vi "DTFDcontroller.vi"() -> ()   [LabVIEW 2020]
uses:
  <vilib>/rvi/Analysis/control/linear/templates/niFPGA FXP Transfer Function Model.ctl
  <vilib>/Platform/TimedLoop/XDataNode/timing_clust.ctl
  <vilib>/Platform/TimedLoop/XDataNode/nitl_modes.ctl
  <vilib>/Platform/TimedLoop/XDataNode/wakeup.ctl
  <vilib>/rvi/Emulation/niFpgaSctlEmulationGetInTimedLoop.vi
  <vilib>/rvi/Emulation/niFpgaEmulationReportErrorSimple.vi
  <vilib>/rvi/Emulation/niFpgaGetClockAttributes.vi
  <vilib>/rvi/Emulation/niFpgaCriticalErrorInLSC.vi
  <vilib>/Platform/TimedLoop/XDataNode/XDataNode.xnode
  <vilib>/Platform/TimedLoop/XDataNode/XDNodeRunTimeDep.lvlib
panel:
  in  "H2 coefficients":T1={"Numerator"=[0.0, 0.0, 0.0, 0.0, 0.0, 0.0, 0.0, 0.0, 0.0], "Denominator"=[0.0, 0.0, 0.0, 0.0, 0.0, 0.0, 0.0, 0.0, 0.0], "Order"=0}
  in  "H1 coefficients":T1={"Numerator"=[0.0, 0.0, 0.0, 0.0, 0.0, 0.0, 0.0, 0.0, 0.0], "Denominator"=[0.0, 0.0, 0.0, 0.0, 0.0, 0.0, 0.0, 0.0, 0.0], "Order"=0}
  in  "KiTs":fxp<+,11,-22>=1.25030055642128e-07 format="%#_61g"
  in  "Kp":fxp<+/-,32,-4>
  in  "min":fxp<+/-,15,-7>=-0.003301858901977539 format="%#_50g"
  in  "max":fxp<+,15,-8>=0.00330197811126709 format="%#_51g"
  in  "Kp_Spool_2":fxp<+,3,4>=10.0 format="%#_20g"
  out "I_cmd":fxp<+/-,40,16>
  in  "meas_rad":fxp<+/-,32,-4>
  in  "ref_rad":fxp<+/-,32,-4>
  in  "Kp_Spool_1":fxp<+,10,14>=10000.0 format="%#_20g"
  in  "meas_spool":fxp<+/-,32,-6>
  in  "reset":bool
  in  "K_OL_RadSpool":fxp<+/-,10,-1>=0.14013671875 format="%#_64g"
  # "PI coefficients"
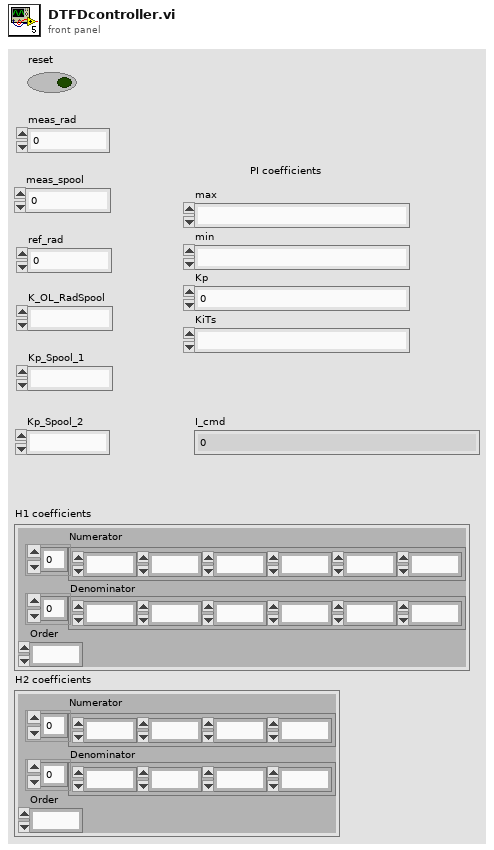
[diagram p1: front panel]
types:
  T1 = typedef "niFPGA FXP Transfer Function Model.ctl" = cluster{"Numerator":fxp<+/-,32,12>[], "Denominator":fxp<+/-,32,12>[], "Order":u8}
  T2 = typedef "XDNodeRunTimeDep.lvlib/timing_clust.ctl" = cluster{"Expected End [f-1]":u64, "Actual End [f-1]":u64, "Finished Late? [f-1]":bool, "Expected End [i-1]":u64, "Actual End [i-1]":u64, "Finished Late? [i-1]":bool, "Expected Start [i]":u64, "Actual Start [i]":u64, "Expected Start [f]":u64, "Actual Start [f]":u64, "Source Name":string, "Structure Name":string, "Period":i64, "Deadline":i64, "Offset":i64, "Start":i64, "Priority":i32, "Timeout":i32, "Mode":T3, "Wakeup Reason":T4, "Error":errorcluster, "Source Type":string, "Secondary Source Type":string, "Global End Time":u64, "Global Start Time":u64, "Frame Duration":u64, "Iteration Duration":u64, "Assigned CPU":i32, "I/O Scan Engine Mode":u32}
  T3 = typedef "XDNodeRunTimeDep.lvlib/nitl_modes.ctl" = enum32{"No Change", "Process missed periods, maintain original phase", "Discard missed periods, maintain original phase", "Process missed periods, ignore original phase", "Discard missed periods, ignore original phase"}
  T4 = typedef "XDNodeRunTimeDep.lvlib/wakeup.ctl" = enum32{"Normal", "Aborted", "Asynchronous wakeup", "Timing source error", "Timed loop error", "Timeout"}
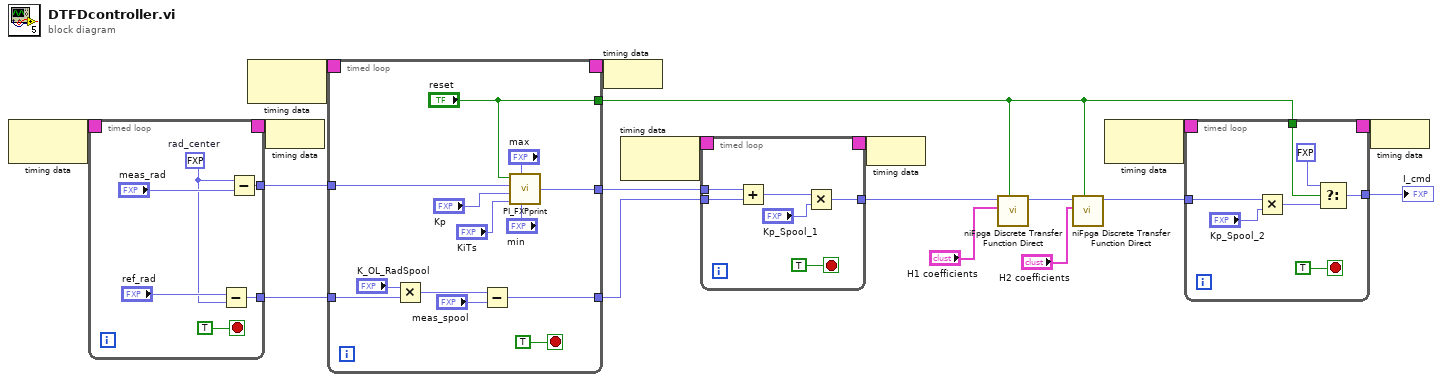
[diagram p0: block diagram]
diagram:
  n1 = node-c288() -> (w15:T2)  [unwired: 1 in]
  n2 = timed-loop {
    timing: w15 -> [_]
    timing-out: [_] -> w14
    tunnel: [w24] -> w11
    tunnel: [w20] -> w10
    stop <- TRUE stop-if-true
    w21 = fxp<+/-,1,1> 0.0  # rad_center
    n3 = Subtract(x="ref_rad", y=w21) -> (x-y=w20:fxp<+/-,32,-4>)
    n4 = Subtract(x=w21, y="meas_rad") -> (x-y=w24:fxp<+/-,32,-4>)
  }
  n5 = node-c288() -> (w19:T2)  [unwired: 1 in]
  n6 = node-c288(w14) -> ()
  n7 = timed-loop {
    timing: w19 -> [_]
    timing-out: [_] -> w18
    tunnel: [w36] -> w12
    tunnel: [w34] -> w13
    tunnel: ["reset"] -> w3
    tunnel: w11 -> [w32]
    tunnel: w10 -> [w35]
    stop <- TRUE stop-if-true
    n8 = Multiply(x="K_OL_RadSpool", y=w35) -> (x*y=w38:fxp<+/-,32,-7>)
    n9 = Subtract(x=w38, y="meas_spool") -> (x-y=w36:fxp<+/-,34,-6>)
    n10 = call "PI_FXPprint.vi"("min"="min", "max"="max", "KiTs"="KiTs", "Kp"="Kp", "e[k]"=w32, "reset"="reset") -> ("u[k]"=w34:fxp<+/-,47,-5>)
  }
  n11 = node-c288(w18) -> ()
  n12 = node-c288() -> (w17:T2)  [unwired: 1 in]
  n13 = timed-loop {
    timing: w17 -> [_]
    timing-out: [_] -> w16
    tunnel: w13 -> [w45]
    tunnel: w12 -> [w44]
    tunnel: [w43] -> w4
    stop <- TRUE stop-if-true
    n14 = Add(x=w45, y=w44) -> (x+y=w48:fxp<+/-,48,-4>)
    n15 = Multiply(x=w48, y="Kp_Spool_1") -> (x*y=w43:fxp<+/-,32,8>)
  }
  n16 = node-c288(w16) -> ()
  n17 = call <vilib>:"niFpga Discrete Transfer Function Direct.vi"("reset"=w3, "FXP Transfer Function Model"="H1 coefficients", "input u(k)"=w4) -> ("output y(k)"=w6:fxp<+/-,32,16>)  [unwired: 8 in]
  n18 = call <vilib>:"niFpga Discrete Transfer Function Direct.vi"("reset"=w3, "FXP Transfer Function Model"="H2 coefficients", "input u(k)"=w6) -> ("output y(k)"=w5:fxp<+/-,32,16>)  [unwired: 8 in]
  n19 = node-c288() -> (w9:T2)  [unwired: 1 in]
  n20 = timed-loop {
    timing: w9 -> [_]
    timing-out: [_] -> w8
    tunnel: [w57] -> w7
    tunnel: w3 -> [w55]
    tunnel: w5 -> [w53]
    stop <- TRUE stop-if-true
    n21 = Multiply(x=w53, y="Kp_Spool_2") -> (x*y=w52:fxp<+/-,32,8>)
    n22 = Select(t=fxp<+/-,40,16> 0.0, s=w55, f=w52) -> (s? t:f=w57:fxp<+/-,40,16>)
  }
  "I_cmd" <- w7
  n23 = node-c288(w8) -> ()
